vi "Conv_Heading_AngleRadians.vi"(10 "Heading":dbl) -> (2 "AngleRadians":dbl)   [LabVIEW 2019, in "PathExecution_Library.lvlib"]
doc: "Convert angle (radians) to heading (+/- PI ) (radians)\nNOTE: increases counter clockwise"
uses:
  PathExecution_Library.lvlib
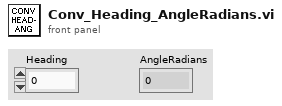
[diagram p1: front panel]
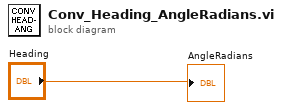
[diagram p0: block diagram]
diagram:
  "AngleRadians" <- "Heading"
